vi "Mic_Close.vi"(8 "error in (no error)":errorcluster, 11 "DAQ Prams":T2={"task ID"=0, "Num Pts"=0, "timeout"=0.0, "FIFO"=0, "Double Bounce"=1.0} {"Double Bounce" format="%#.2g"; "task ID" format="%.0x"}) -> (0 "error out":errorcluster)   [LabVIEW 2022 SP3]
uses:
  <vilib>/sound2/lvsound2.llb/Sound Input Task ID.ctl
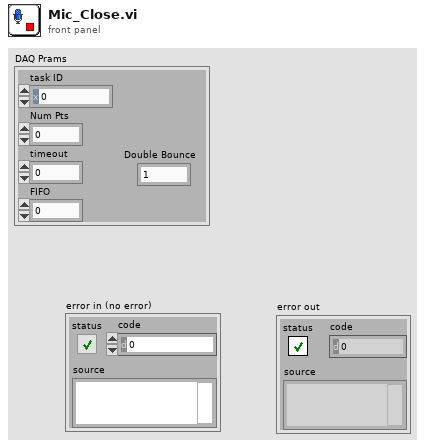
[diagram p1: front panel]
types:
  T1 = typedef "Sound Input Task ID.ctl" = u32
  T2 = cluster{"task ID":T1, "Num Pts":i32, "timeout":dbl, "FIFO":i32, "Double Bounce":dbl}
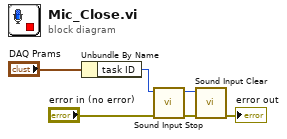
[diagram p0: block diagram]
diagram:
  n1 = Unbundle By Name("DAQ Prams") -> ("task ID"=w5:T1)
  n2 = call <vilib>:"Sound Input Stop.vi"("error in (no error)"="error in (no error)", "task ID"=w5) -> ("error out"=w2:errorcluster, "task ID out"=w3:T1)  [unwired: 8 in]
  n3 = call <vilib>:"Sound Input Clear.vi"("error in (no error)"=w2, "task ID"=w3) -> ("error out"=→"error out":errorcluster)  [unwired: 9 in]
